vi "vision_acquisition.vi"() -> ()   [LabVIEW 2011]
panel:
  in  "Number of Images":i32=4
  out "Image Out":T1(plugin-control)
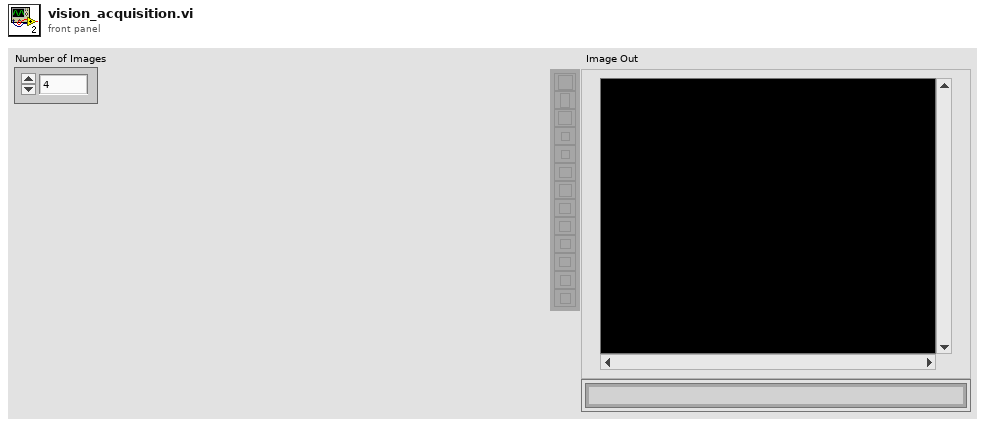
[diagram p1: front panel]
types:
  T1 = typedef "IMAQ Image.ctl" = refnum<image>
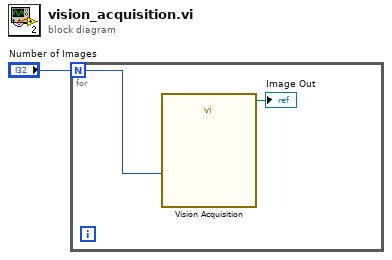
[diagram p0: block diagram]
diagram:
  n1 = for {
    N: "Number of Images" -> [w2]
    n2 = call "Vision Acquisition"("Number of Images"=w2) -> ("Image Out"=→"Image Out":T1)  [unwired: 24 in, 2 out]
  }
